vi "SWS.vi"(8 "Stopp":bool, 10 "SLOT":i32=100 min=0 max=999 step=100 format="%03d", 11 "USB":i32) -> ()   [LabVIEW 2020]
doc: "This VI provides a GUI for SWS modules. It implements an abstract module interface, where callers provide the only necessary and sufficient information for callee modules via the datafields USB, SLOT and Stopp. All module intern information are handled hidden by the module. Thereby, a caller must not \"know\" about such internals."
uses:
  <vilib>/Platform/TimedLoop/XDataNode/timing_clust.ctl
  <vilib>/Platform/TimedLoop/XDataNode/nitl_modes.ctl
  <vilib>/Platform/TimedLoop/XDataNode/wakeup.ctl
  <vilib>/platform/TimedLoop/XDataNode/XDataNode.xnode
  <vilib>/Platform/TimedLoop/XDataNode/XDNodeRunTimeDep.lvlib
panel:
  in  "BeamPosVert":i16(slide) caption="Vertical" min=0 max=0 scale=0.0..1.0
  in  "BeamPosHoriz":i16(slide) caption="Horizontal" min=0 max=0 scale=0.0..1.0
  out "Laser Intensity":sgl caption="a.u." format="%.1f"
  in  "Bypass Filter":bool
  in  "Bandwidth":sgl(slide)=3.0 min=0 max=3 scale=0.0..1.0
  in  "Center Wavelength":sgl(slide)=480.0 min=0 max=500 scale=0.0..1.0
  # "Beam Coupling Position:"
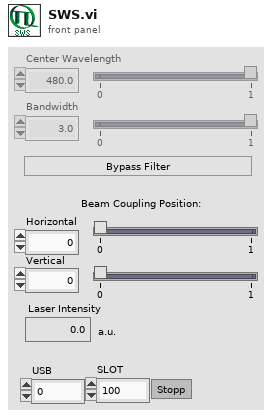
[diagram p1: front panel]
types:
  T1 = typedef "XDNodeRunTimeDep.lvlib/timing_clust.ctl" = cluster{"Expected End [f-1]":u64, "Actual End [f-1]":u64, "Finished Late? [f-1]":bool, "Expected End [i-1]":u64, "Actual End [i-1]":u64, "Finished Late? [i-1]":bool, "Expected Start [i]":u64, "Actual Start [i]":u64, "Expected Start [f]":u64, "Actual Start [f]":u64, "Source Name":string, "Structure Name":string, "Period":i64, "Deadline":i64, "Offset":i64, "Start":i64, "Priority":i32, "Timeout":i32, "Mode":T2, "Wakeup Reason":T3, "Error":errorcluster, "Source Type":string, "Secondary Source Type":string, "Global End Time":u64, "Global Start Time":u64, "Frame Duration":u64, "Iteration Duration":u64, "Assigned CPU":i32, "I/O Scan Engine Mode":u32}
  T2 = typedef "XDNodeRunTimeDep.lvlib/nitl_modes.ctl" = enum32{"No Change", "Process missed periods, maintain original phase", "Discard missed periods, maintain original phase", "Process missed periods, ignore original phase", "Discard missed periods, ignore original phase"}
  T3 = typedef "XDNodeRunTimeDep.lvlib/wakeup.ctl" = enum32{"Normal", "Aborted", "Asynchronous wakeup", "Timing source error", "Timed loop error", "Timeout"}
  T4 = cluster{"UpperWL":u32, "LowerWL":u32, "IncrWL":u32, "PPMToggleWL":u32, "UpperBW":u32, "LowerBW":u32, "IncrBW":u32, "UpperBeamPos":i32, "LowerBeamPos":i32, "IncrBeamPos":i32}
  T5 = enum8{"Enabled", "Disabled", "Disabled and Grayed Out"}
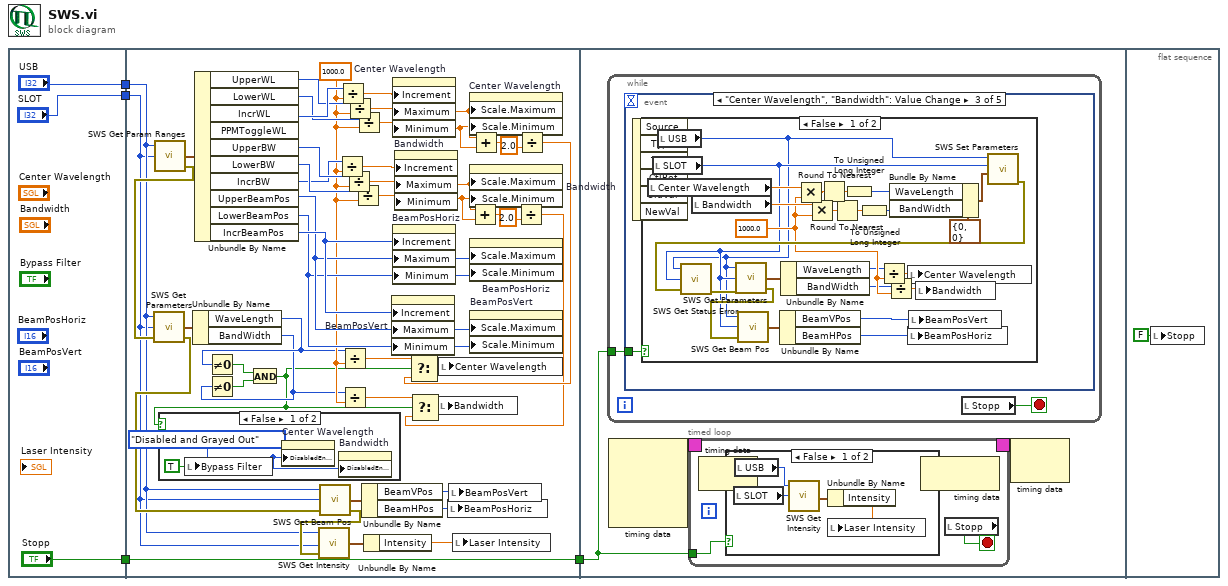
[diagram p0: block diagram]
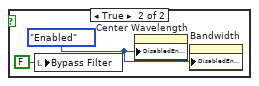
[diagram p2: hidden frame]
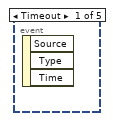
[diagram p4: hidden frame]
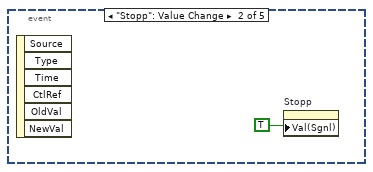
[diagram p5: hidden frame]
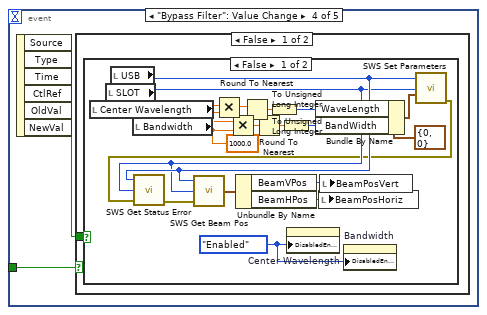
[diagram p7: hidden frame]
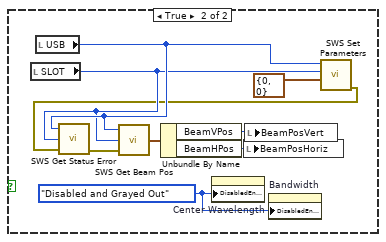
[diagram p8: hidden frame]
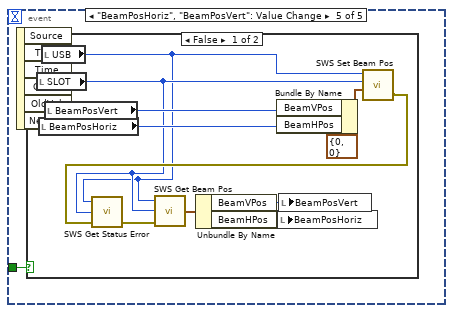
[diagram p10: hidden frame]
diagram:
  n1 = flat-sequence {
    tunnel: ["USB"] -> w4
    tunnel: ["SLOT"] -> w3
    tunnel: ["Stopp"] -> w1
    tunnel: w4 -> [w31]
    tunnel: w3 -> [w30]
    tunnel: [w27] -> w2
    tunnel: w1 -> [w27]
    tunnel: w2 -> [w56]
    frame #0 {
    }
    frame #1 {
      w36 = 1000.0 ("y")
      n2 = call "SWS Get Param Ranges.vi"("SLOT"=w30, "DevIdx"=w31) -> ("error out"=w39:errorcluster, "SWS Param Ranges"=w51:T4)  [unwired: 1 in, 1 out]
      n3 = call "SWS Get Parameters.vi"("error in (no error)"=w39, "SlotId"=w30, "DevIdx"=w31) -> ("error out"=w38:errorcluster, "SWS Parameters"=w37:cluster{"WaveLength":u32, "BandWidth":u32})  [unwired: 1 out]
      n4 = Unbundle By Name(w37) -> ("WaveLength"=w10:u32, "BandWidth"=w9:u32)
      n5 = Unbundle By Name(w51) -> ("UpperWL"=w48:u32, "LowerWL"=w47:u32, "IncrWL"=w49:u32, "UpperBW"=w45:u32, "LowerBW"=w44:u32, "IncrBW"=w43:u32, "UpperBeamPos"=w41:i32, "LowerBeamPos"=w40:i32, "IncrBeamPos"=w42:i32)  [unwired: 1 out]
      n6 = Not Equal To 0?(x=w10) -> (x != 0?=w26:bool)
      n7 = Not Equal To 0?(x=w9) -> (x != 0?=w25:bool)
      n8 = And(x=w26, y=w25) -> (x .and. y?=w8:bool)
      n9 = case shown="False" w8 {
        frame False {
          w53 = T5."Disabled and Grayed Out" ("Disabled")
          n10 = local write "Bypass Filter"(TRUE ("Bypass Filter")) -> ()
          n11 = property on="Center Wavelength" class="Slide (strict)"("DisabledEnum"=w53) -> ()  [unwired: 2 in, 2 out]
          n12 = property on="Bandwidth" class="Slide (strict)"("DisabledEnum"=w53) -> ()  [unwired: 2 in, 2 out]
        }
        frame True {
          w55 = T5."Enabled" ("Disabled")
          n13 = local write "Bypass Filter"(FALSE ("Bypass Filter")) -> ()
          n14 = property on="Center Wavelength" class="Slide (strict)"("DisabledEnum"=w55) -> ()  [unwired: 2 in, 2 out]
          n15 = property on="Bandwidth" class="Slide (strict)"("DisabledEnum"=w55) -> ()  [unwired: 2 in, 2 out]
        }
      }
      n16 = call "SWS Get Beam Pos.vi"("error in (no error)"=w38, "SlotId"=w30, "DevIdx"=w31) -> ("error out"=w32:errorcluster, "SWS Beam Pos"=w35:cluster{"BeamVPos":i16, "BeamHPos":i16})  [unwired: 1 out]
      n17 = call "SWS Get Intensity.vi"("error in (no error)"=w32, "SlotId"=w30, "DevIdx"=w31) -> ("SWS Intensity"=w29:cluster{"IntensityRaw":u32, "Intensity":sgl})  [unwired: 2 out]
      n18 = Divide(x=w43, y=w36) -> (x/y=w46:dbl)
      n19 = Divide(x=w49, y=w36) -> (x/y=w50:dbl)
      n20 = Divide(x=w10, y=w36) -> (x/y=w22:dbl)
      n21 = Divide(x=w9, y=w36) -> (x/y=w21:dbl)
      n22 = Divide(x=w45, y=w36) -> (x/y=w14:dbl)
      n23 = Divide(x=w48, y=w36) -> (x/y=w16:dbl)
      n24 = Divide(x=w44, y=w36) -> (x/y=w13:dbl)
      n25 = Divide(x=w47, y=w36) -> (x/y=w15:dbl)
      n26 = Unbundle By Name(w35) -> ("BeamVPos"=w34:i16, "BeamHPos"=w33:i16)
      n27 = Unbundle By Name(w29) -> ("Intensity"=w28:sgl)
      n28 = property on="BeamPosVert" class="Slide (strict)"("Increment"=w42, "Maximum"=w41, "Minimum"=w40) -> ()  [unwired: 2 in, 2 out]
      n29 = property on="Center Wavelength" class="Slide (strict)"("Increment"=w50, "Maximum"=w16, "Minimum"=w15) -> ()  [unwired: 2 in, 2 out]
      n30 = property on="BeamPosHoriz" class="Slide (strict)"("Increment"=w42, "Maximum"=w41, "Minimum"=w40) -> ()  [unwired: 2 in, 2 out]
      n31 = property on="Bandwidth" class="Slide (strict)"("Increment"=w46, "Maximum"=w14, "Minimum"=w13) -> ()  [unwired: 2 in, 2 out]
      n32 = local write "BeamPosHoriz"(w33) -> ()
      n33 = local write "BeamPosVert"(w34) -> ()
      n34 = local write "Laser Intensity"(w28) -> ()
      n35 = property on="Center Wavelength" class="Slide (strict)"("Scale.Maximum"=w16, "Scale.Minimum"=w15) -> ()  [unwired: 2 in, 2 out]
      n36 = property on="Bandwidth" class="Slide (strict)"("Scale.Maximum"=w14, "Scale.Minimum"=w13) -> ()  [unwired: 2 in, 2 out]
      n37 = Add(x=w14, y=w13) -> (x+y=w20:dbl)
      n38 = property on="BeamPosHoriz" class="Slide (strict)"("Scale.Maximum"=w41, "Scale.Minimum"=w40) -> ()  [unwired: 2 in, 2 out]
      n39 = property on="BeamPosVert" class="Slide (strict)"("Scale.Maximum"=w41, "Scale.Minimum"=w40) -> ()  [unwired: 2 in, 2 out]
      n40 = Add(x=w16, y=w15) -> (x+y=w18:dbl)
      n41 = Divide(x=w20, y=2.0) -> (x/y=w11:dbl)
      n42 = Select(t=w21, s=w8, f=w11) -> (s? t:f=w23:dbl)
      n43 = local write "Bandwidth"(w23) -> ()
      n44 = Divide(x=w18, y=2.0) -> (x/y=w12:dbl)
      n45 = Select(t=w22, s=w8, f=w12) -> (s? t:f=w24:dbl)
      n46 = local write "Center Wavelength"(w24) -> ()
    }
    frame #2 {
      n47 = while {
        tunnel: w56 -> [w69]
        stop <- w70 stop-if-true
        n48 = event shown="[2] \"Center Wavelength\", \"Bandwidth\": Value Change" {
          selector: _ -> [_ _ _ _ _]
          dyn-events: _ -> [_ _ _ _ _]
          timeout: _ -> [_ _ _ _ _]
          tunnel: w69 -> [_ _ w72 w98 w128]
          event Timeout {
            n49 = event-data() -> ()  [unwired: 1 in, 3 out]
          }
          event "Stopp": Value Change {
            n50 = event-data() -> ()  [unwired: 1 in, 6 out]
            n51 = property on="Stopp" class="Bool (strict)"("Val(Sgnl)"=TRUE) -> ()  [unwired: 2 in, 2 out]
          }
          event "Center Wavelength", "Bandwidth": Value Change {
            n52 = event-data() -> ()  [unwired: 1 in, 6 out]
            n53 = case shown="False" w72 {
              frame False {
                w81 = sgl 1000.0 ("Bandwidth")
                n54 = local read "Center Wavelength"() -> (w94:sgl)
                n55 = local read "SLOT"() -> (w74:i32)
                n56 = local read "USB"() -> (w73:i32)
                n57 = local read "Bandwidth"() -> (w93:sgl)
                n58 = Multiply(x=w94, y=w81) -> (x*y=w92:sgl)
                n59 = Multiply(x=w93, y=w81) -> (x*y=w91:sgl)
                n60 = Round To Nearest(number=w92) -> (nearest integer value=w90:sgl)
                n61 = Round To Nearest(number=w91) -> (nearest integer value=w89:sgl)
                n62 = To Unsigned Long Integer(number=w90) -> (unsigned 32bit integer=w87:u32)
                n63 = To Unsigned Long Integer(number=w89) -> (unsigned 32bit integer=w88:u32)
                n64 = Bundle By Name(cluster=cluster{"WaveLength":u32, "BandWidth":u32} {"WaveLength"=0, "BandWidth"=0} ("SWS Parameters"), "WaveLength"=w87, "BandWidth"=w88) -> (w95:cluster{"WaveLength":u32, "BandWidth":u32})
                n65 = call "SWS Set Parameters.vi"("SWS Parameters"=w95, "SlotId"=w74, "DevIdx"=w73) -> ("error out"=w85:errorcluster)  [unwired: 3 in, 1 out]
                n66 = call "SWS Get Status Error.vi"("iDevIdx"=w73, "SLOT"=w74, "error in (no error)"=w85) -> ("error out"=w76:errorcluster)  [unwired: 3 out]
                n67 = call "SWS Get Parameters.vi"("error in (no error)"=w76, "SlotId"=w74, "DevIdx"=w73) -> ("error out"=w75:errorcluster, "SWS Parameters"=w82:cluster{"WaveLength":u32, "BandWidth":u32})  [unwired: 1 out]
                n68 = call "SWS Get Beam Pos.vi"("error in (no error)"=w75, "SlotId"=w74, "DevIdx"=w73) -> ("SWS Beam Pos"=w86:cluster{"BeamVPos":i16, "BeamHPos":i16})  [unwired: 2 out]
                n69 = Unbundle By Name(w86) -> ("BeamVPos"=w84:i16, "BeamHPos"=w83:i16)
                n70 = Unbundle By Name(w82) -> ("WaveLength"=w79:u32, "BandWidth"=w80:u32)
                n71 = Divide(x=w79, y=w81) -> (x/y=w78:sgl)
                n72 = Divide(x=w80, y=w81) -> (x/y=w77:sgl)
                n73 = local write "Center Wavelength"(w78) -> ()
                n74 = local write "BeamPosHoriz"(w83) -> ()
                n75 = local write "BeamPosVert"(w84) -> ()
                n76 = local write "Bandwidth"(w77) -> ()
              }
              frame True {
              }
            }
          }
          event "Bypass Filter": Value Change {
            n77 = event-data() -> ("NewVal"=w97:bool)  [unwired: 1 in, 5 out]
            n78 = case shown="False" w98 {
              tunnel: w97 -> [w99 _]
              frame False {
                n79 = case shown="False" w99 {
                  frame False {
                    w105 = sgl 1000.0 ("Bandwidth")
                    w111 = T5."Enabled" ("Disabled")
                    n80 = local read "Center Wavelength"() -> (w101:sgl)
                    n81 = local read "SLOT"() -> (w116:i32)
                    n82 = local read "USB"() -> (w117:i32)
                    n83 = local read "Bandwidth"() -> (w100:sgl)
                    n84 = Multiply(x=w101, y=w105) -> (x*y=w102:sgl)
                    n85 = Multiply(x=w100, y=w105) -> (x*y=w108:sgl)
                    n86 = Round To Nearest(number=w102) -> (nearest integer value=w107:sgl)
                    n87 = Round To Nearest(number=w108) -> (nearest integer value=w106:sgl)
                    n88 = To Unsigned Long Integer(number=w107) -> (unsigned 32bit integer=w103:u32)
                    n89 = To Unsigned Long Integer(number=w106) -> (unsigned 32bit integer=w104:u32)
                    n90 = property on="Center Wavelength" class="Slide (strict)"("DisabledEnum"=w111) -> ()  [unwired: 2 in, 2 out]
                    n91 = Bundle By Name(cluster=cluster{"WaveLength":u32, "BandWidth":u32} {"WaveLength"=0, "BandWidth"=0} ("SWS Parameters"), "WaveLength"=w103, "BandWidth"=w104) -> (w109:cluster{"WaveLength":u32, "BandWidth":u32})
                    n92 = property on="Bandwidth" class="Slide (strict)"("DisabledEnum"=w111) -> ()  [unwired: 2 in, 2 out]
                    n93 = call "SWS Set Parameters.vi"("SWS Parameters"=w109, "SlotId"=w116, "DevIdx"=w117) -> ("error out"=w113:errorcluster)  [unwired: 3 in, 1 out]
                    n94 = call "SWS Get Status Error.vi"("iDevIdx"=w117, "SLOT"=w116, "error in (no error)"=w113) -> ("error out"=w118:errorcluster)  [unwired: 3 out]
                    n95 = call "SWS Get Beam Pos.vi"("error in (no error)"=w118, "SlotId"=w116, "DevIdx"=w117) -> ("SWS Beam Pos"=w112:cluster{"BeamVPos":i16, "BeamHPos":i16})  [unwired: 2 out]
                    n96 = Unbundle By Name(w112) -> ("BeamVPos"=w114:i16, "BeamHPos"=w115:i16)
                    n97 = local write "BeamPosHoriz"(w115) -> ()
                    n98 = local write "BeamPosVert"(w114) -> ()
                  }
                  frame True {
                    w119 = T5."Disabled and Grayed Out" ("Disabled")
                    n99 = local read "SLOT"() -> (w124:i32)
                    n100 = local read "USB"() -> (w125:i32)
                    n101 = property on="Center Wavelength" class="Slide (strict)"("DisabledEnum"=w119) -> ()  [unwired: 2 in, 2 out]
                    n102 = property on="Bandwidth" class="Slide (strict)"("DisabledEnum"=w119) -> ()  [unwired: 2 in, 2 out]
                    n103 = call "SWS Set Parameters.vi"("SWS Parameters"=cluster{"WaveLength":u32, "BandWidth":u32} {"WaveLength"=0, "BandWidth"=0}, "SlotId"=w124, "DevIdx"=w125) -> ("error out"=w121:errorcluster)  [unwired: 3 in, 1 out]
                    n104 = call "SWS Get Status Error.vi"("iDevIdx"=w125, "SLOT"=w124, "error in (no error)"=w121) -> ("error out"=w127:errorcluster)  [unwired: 3 out]
                    n105 = call "SWS Get Beam Pos.vi"("error in (no error)"=w127, "SlotId"=w124, "DevIdx"=w125) -> ("SWS Beam Pos"=w120:cluster{"BeamVPos":i16, "BeamHPos":i16})  [unwired: 2 out]
                    n106 = Unbundle By Name(w120) -> ("BeamVPos"=w122:i16, "BeamHPos"=w123:i16)
                    n107 = local write "BeamPosHoriz"(w123) -> ()
                    n108 = local write "BeamPosVert"(w122) -> ()
                  }
                }
              }
              frame True {
              }
            }
          }
          event "BeamPosHoriz", "BeamPosVert": Value Change {
            n109 = event-data() -> ()  [unwired: 1 in, 6 out]
            n110 = case shown="False" w128 {
              frame False {
                n111 = local read "SLOT"() -> (w130:i32)
                n112 = local read "BeamPosHoriz"() -> (w134:i16)
                n113 = local read "USB"() -> (w129:i32)
                n114 = local read "BeamPosVert"() -> (w135:i16)
                n115 = Bundle By Name(cluster=cluster{"BeamVPos":i16, "BeamHPos":i16} {"BeamVPos"=0, "BeamHPos"=0} ("SWS Beam Pos"), "BeamVPos"=w135, "BeamHPos"=w134) -> (w132:cluster{"BeamVPos":i16, "BeamHPos":i16})
                n116 = call "SWS Set Beam Pos.vi"("SWS Beam Pos"=w132, "SlotId"=w130, "DevIdx"=w129) -> ("error out"=w131:errorcluster)  [unwired: 1 in, 1 out]
                n117 = call "SWS Get Status Error.vi"("iDevIdx"=w129, "SLOT"=w130, "error in (no error)"=w131) -> ("error out"=w133:errorcluster)  [unwired: 3 out]
                n118 = call "SWS Get Beam Pos.vi"("error in (no error)"=w133, "SlotId"=w130, "DevIdx"=w129) -> ("SWS Beam Pos"=w139:cluster{"BeamVPos":i16, "BeamHPos":i16})  [unwired: 2 out]
                n119 = Unbundle By Name(w139) -> ("BeamVPos"=w138:i16, "BeamHPos"=w137:i16)
                n120 = local write "BeamPosHoriz"(w137) -> ()
                n121 = local write "BeamPosVert"(w138) -> ()
              }
              frame True {
              }
            }
          }
        }
        n122 = local read "Stopp"() -> (w70:bool)
      }
      n123 = node-c288() -> (w58:T1)  [unwired: 4 in]
      n124 = timed-loop {
        timing: w58 -> [_]
        timing-out: [_] -> w57
        tunnel: w56 -> [w59]
        stop <- w60 stop-if-true
        n125 = node-c288() -> ()  [unwired: 1 in, 1 out]
        n126 = case shown="False" w59 {
          frame False {
            n127 = local read "SLOT"() -> (w61:i32)
            n128 = local read "USB"() -> (w62:i32)
            n129 = call "SWS Get Intensity.vi"("SlotId"=w61, "DevIdx"=w62) -> ("SWS Intensity"=w63:cluster{"IntensityRaw":u32, "Intensity":sgl})  [unwired: 1 in, 2 out]
            n130 = Unbundle By Name(w63) -> ("Intensity"=w64:sgl)
            n131 = local write "Laser Intensity"(w64) -> ()
          }
          frame True {
          }
        }
        n132 = node-c288() -> ()  [unwired: 1 in, 1 out]
        n133 = local read "Stopp"() -> (w60:bool)
      }
      n134 = node-c288(w57) -> ()  [unwired: 1 out]
    }
    frame #3 {
      n135 = local write "Stopp"(FALSE ("Stopp")) -> ()
    }
  }
